vi "ActFollowAbsoluteTrajectory.vi"(10 "Trajectory":T1 {"States"."POSE"."ROTATION"."SIN" format="%13.4f"; "States"."POSE"."ROTATION"."COS" format="%13.4f"; "States"."POSE"."ROTATION"."VALUE" format="%13.4f"; "States"."POSE"."TRANSLATION"."Y" format="%14.3f"; "States"."POSE"."TRANSLATION"."X" format="%14.3f"; "TotalTImeSecs" format="%20.3f"}, 11 "FirstTime":bool) -> (1 "Done":bool, 2 "RightSpeed":dbl, 3 "LeftSpeed":dbl)   [LabVIEW 2020]
uses:
  <vilib>/Rock Robotics/WPI/ThirdParty/JAS_Junk/TrajLib/Trajectory_Library.lvlib
  <vilib>/Rock Robotics/WPI/ThirdParty/JAS_Junk/TrajLib/TypeDef/TRANSLATION2D.ctl
  <vilib>/Rock Robotics/WPI/ThirdParty/JAS_Junk/TrajLib/TypeDef/ROTATION2D.ctl
  <vilib>/Rock Robotics/WPI/ThirdParty/JAS_Junk/TrajLib/TypeDef/POSE2D.ctl
  <vilib>/Rock Robotics/WPI/ThirdParty/JAS_Junk/TrajLib/TypeDef/TRAJ_STATE.ctl
  <vilib>/Rock Robotics/WPI/ThirdParty/JAS_Junk/TrajLib/TypeDef/TRAJECTORY.ctl
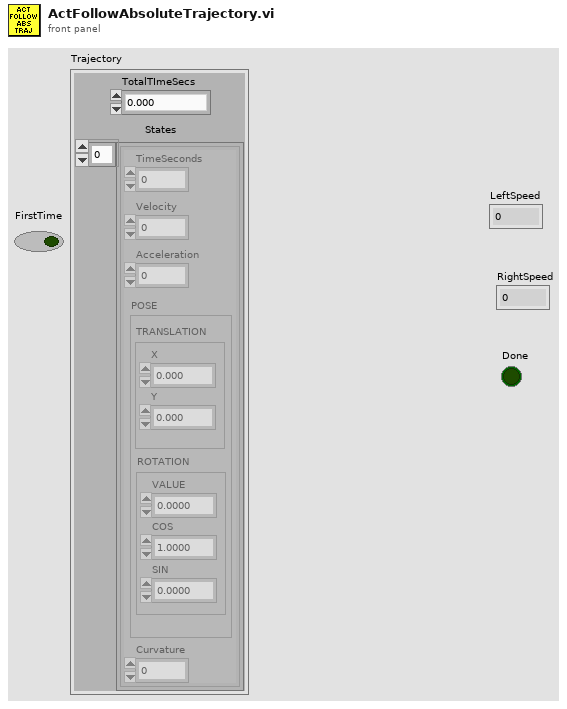
[diagram p1: front panel]
types:
  T1 = typedef "Trajectory_Library.lvlib/TRAJECTORY.ctl" = cluster{"TotalTImeSecs":dbl, "States":T2[]}
  T2 = typedef "Trajectory_Library.lvlib/TRAJ_STATE.ctl" = cluster{"TimeSeconds":dbl, "Velocity":dbl, "Acceleration":dbl, "POSE":T3, "Curvature":dbl}
  T3 = typedef "Trajectory_Library.lvlib/POSE2D.ctl" = cluster{"TRANSLATION":T4, "ROTATION":T5}
  T4 = typedef "Trajectory_Library.lvlib/TRANSLATION2D.ctl" = cluster{"X":dbl, "Y":dbl}
  T5 = typedef "Trajectory_Library.lvlib/ROTATION2D.ctl" = cluster{"VALUE":dbl, "COS":dbl, "SIN":dbl}
  T6 = typedef "Trajectory_Library.lvlib/RAMSETE_EXE_TUNING.ctl" = cluster{"B":dbl, "Zeta":dbl, "X Tolerance M":dbl, "Y Tolerance M":dbl, "Heading Tolerance RAD":dbl, "Track Width M":dbl, "Max Speed M/S":dbl}
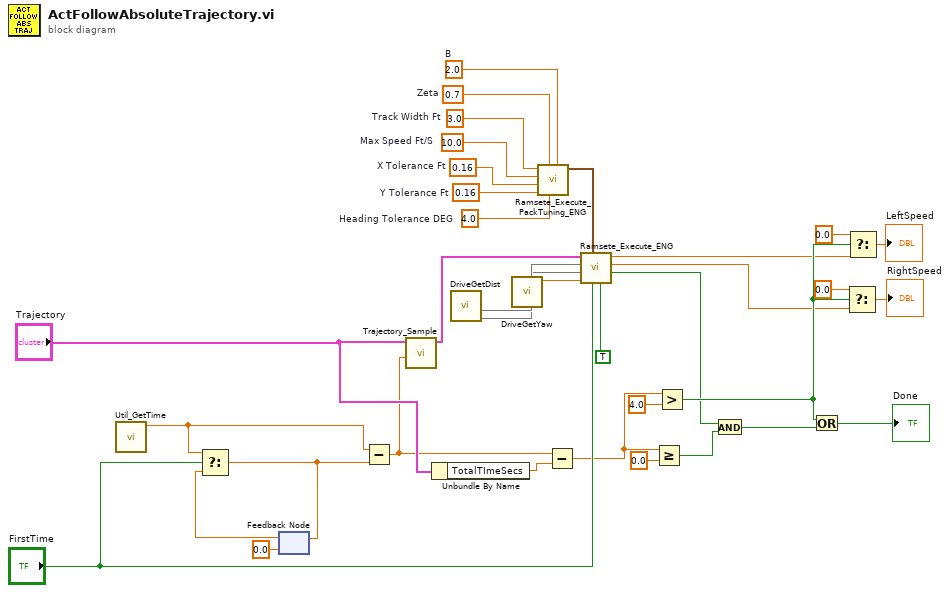
[diagram p0: block diagram]
diagram:
  w35 = 3.0  # Track Width Ft
  w34 = 10.0  # Max Speed Ft/S
  w33 = 0.16  # X Tolerance Ft
  w32 = 0.16  # Y Tolerance Ft
  w31 = 0.7  # Zeta
  w30 = 4.0  # Heading Tolerance DEG
  w29 = 2.0  # B
  n1 = call <vilib>:"Util_GetTime.vi"() -> ("FPGA_Time_Seconds"=w20:dbl)  [unwired: 9 in, 2 out]
  n2 = feedback #1(0.0) -> (w22:dbl)
  n3 = Select(t=w20, s="FirstTime", f=w22) -> (s? t:f=w19:dbl)
  n4 = feedback-in #1(w19) -> ()
  n5 = Subtract(x=w20, y=w19) -> (x-y=w16:dbl)
  n6 = call <vilib>:"Trajectory_Sample.vi"("Time"=w16, "InputTRAJECTORY"="Trajectory") -> ("OutputTRAJ_STATE"=w26:T2)  [unwired: 9 in]
  n7 = Unbundle By Name("Trajectory") -> ("TotalTImeSecs"=w15:dbl)
  n8 = call "DriveGetDist.vi"() -> (0:w24, 1:w25)  [unwired: 9 in, 1 out]
  n9 = call "DriveGetYaw.vi"() -> ("Yaw"=w23:dbl)  [unwired: 11 in]
  n10 = call <vilib>:"Ramsete_Execute_PackTuning_ENG.vi"("B"=w29, "Heading Tolerance DEG"=w30, "Zeta"=w31, "Y Tolerance Ft"=w32, "X Tolerance Ft"=w33, "Max Speed Ft/S"=w34, "Track Width Ft"=w35) -> ("RAMSETE_EXE_TUNING"=w28:T6)  [unwired: 4 in]
  n11 = Subtract(x=w16, y=w15) -> (x-y=w7:dbl)
  n12 = call <vilib>:"Ramsete_Execute_ENG.vi"("Enabled"=TRUE, "Reset"="FirstTime", "RAMSETE_EXE_TUNING"=w28, "Gyro-Deg\n(Inc counterclockwise)"=w23, "RightDist-Ft"=w24, "LeftDist-Ft"=w25, "TRAJ_STATE  SI"=w26) -> ("AtReference"=w5:bool, "Right Speed Dmd Ft/S"=w3:dbl, "Left Speed Dmd Ft/S"=w4:dbl)  [unwired: 2 out]
  n13 = Greater Or Equal?(x=w7, y=0.0) -> (x >= y?=w6:bool)
  n14 = Greater?(x=w7, y=4.0) -> (0:w10:bool)
  n15 = And(x=w5, y=w6) -> (x .and. y?=w13:bool)
  n16 = Or(x=w10, y=w13) -> (x .or. y?=→"Done":bool)
  n17 = Select(t=0.0, s=w10, f=w3) -> (s? t:f=→"RightSpeed":dbl)
  n18 = Select(t=0.0, s=w10, f=w4) -> (s? t:f=→"LeftSpeed":dbl)
